vi "X_gConstraintsFun.vi"() -> (0 "constraints cluster":T1)   [LabVIEW 2019]
panel:
  in  "Ts":dbl=0.001
  in  "w0":dbl=1.0
  in  "weight":dbl[](array[numeric])=[1e-06, 1e-06, 1e-06, 1e-06, 1e-06, 1e-06, 1e-06, 1e-06, 1e-06, 1e-06, 1e-06, 1e-06, 1e-06, 1e-06, 1e-06, 1e-06, 1e-06, 1e-06]
  out "gamma":cdb
  out "beta":cdb[](array[numeric])
  in  "Ki":dbl[](array[numeric])=[1000.0, 100.0, 10.0, 1.4, 0.831, 0.35, 0.143, 0.139, 0.131, 0.113, 0.102, 0.092, 0.083, 0.0, 0.0, 0.0, 0.0, 0.0]
  out "OmegaC":dbl[](array[numeric])
  in  "freq(Hz)":dbl[](array[numeric])=[0.1, 1.0, 10.0, 100.0, 325.0, 500.0, 700.0, 1000.0, 1322.0, 1800.0, 2200.0, 2600.0, 3000.0, 0.0, 0.0, 0.0, 0.0, 0.0]
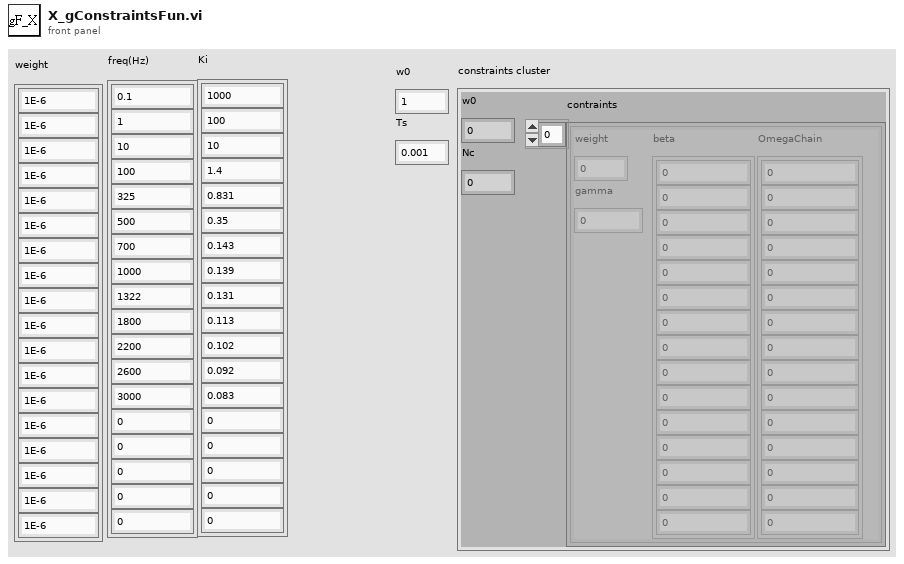
[diagram p1: front panel]
types:
  T1 = cluster{"w0":dbl, "contraints":cluster{"beta":dbl[], "gamma":dbl, "OmegaChain":dbl[], "weight":dbl}[], "Nc":i32}
  T2 = cluster{"v2p.num":dbl[], ".v2p.den":dbl[], "N.num":dbl[], "M.num":dbl[], "X.num":dbl[], "W.num":dbl[], "N.den":dbl[], "W.den":dbl[], "M.den":dbl[], "X.den":dbl[]}
  T3 = cluster{"beta":dbl[], "gamma":dbl, "OmegaChain":dbl[], "weight":dbl}
  T4 = cluster{"v2p":cdb, "N":cdb, "M":cdb, ".X":cdb, "W":cdb}
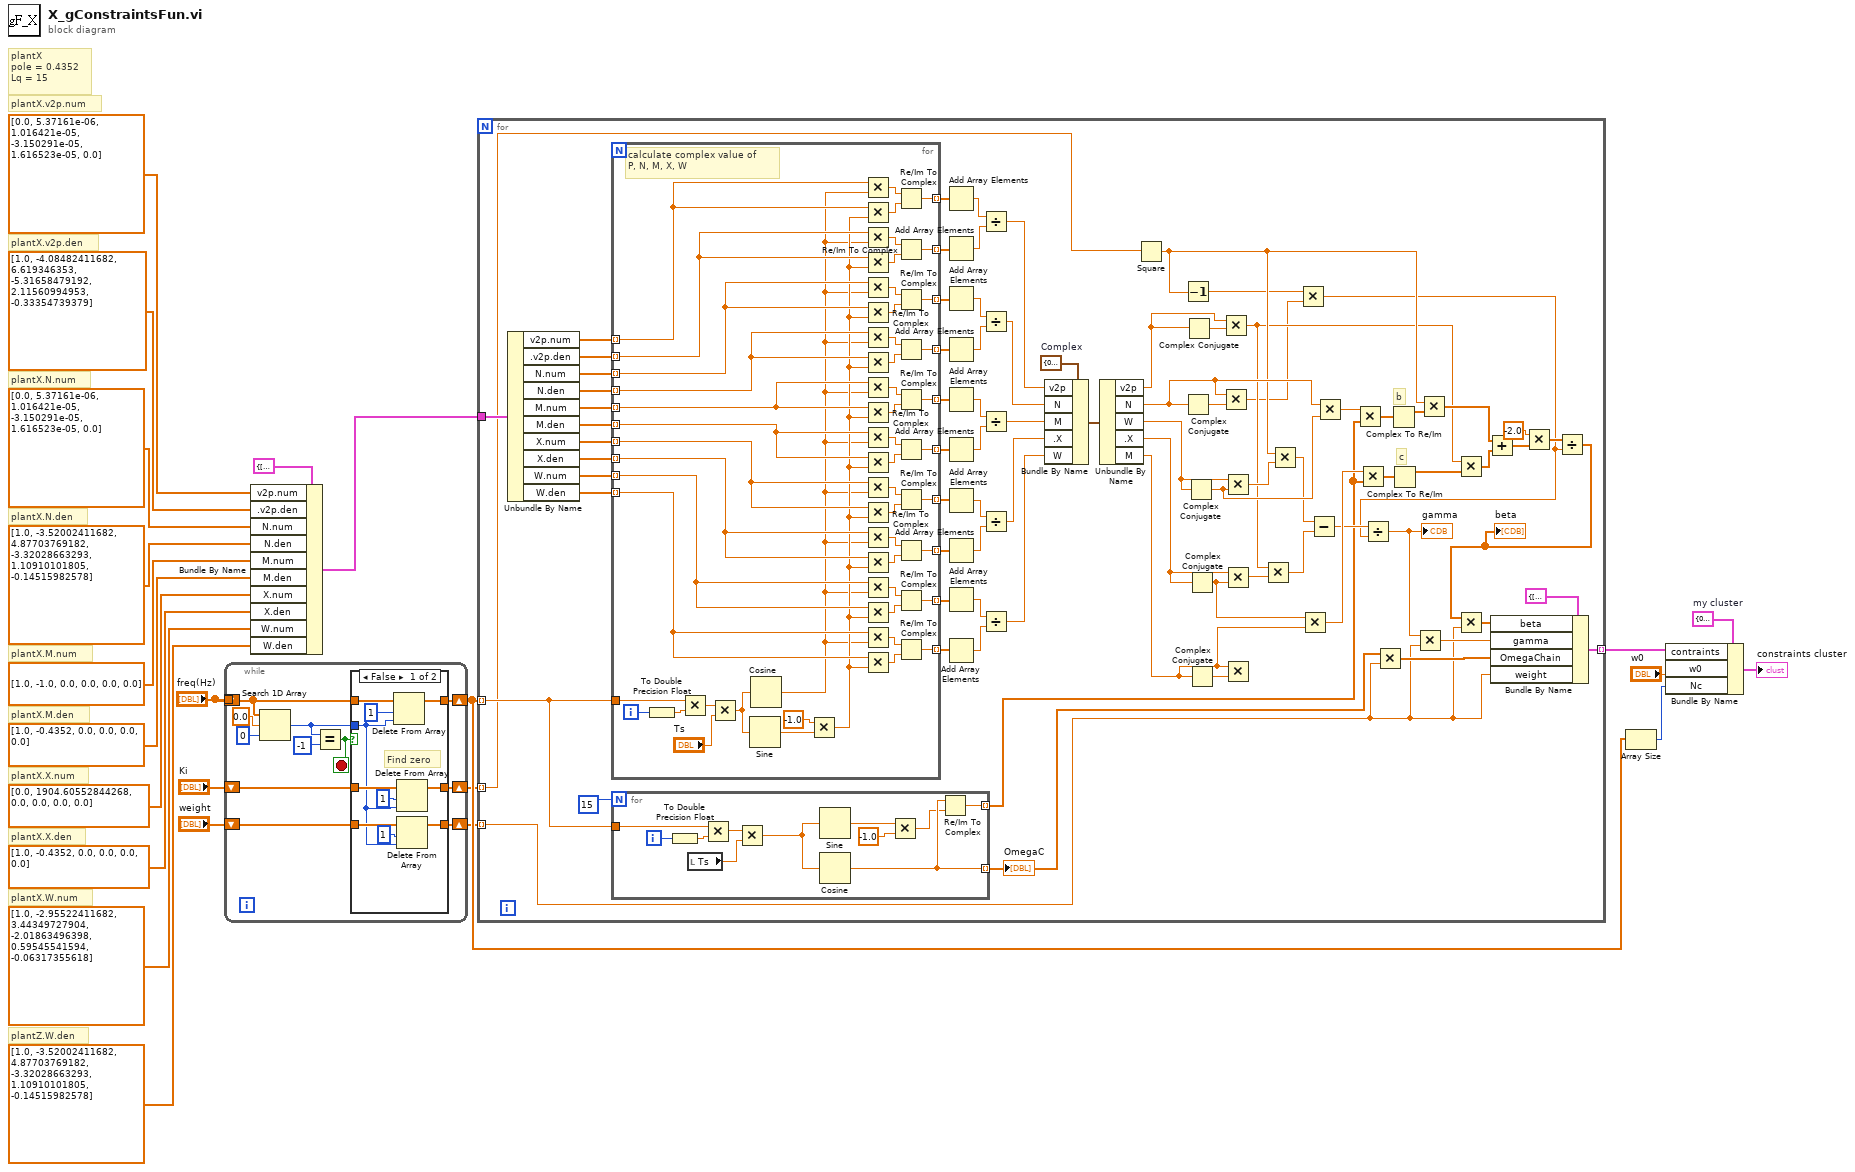
[diagram p0: block diagram]
diagram:
  w21 = T1 {"w0"=0.0, "contraints"=[], "Nc"=0}  # my cluster
  # "plantX.N.den"
  # "plantZ.W.den"
  # "plantX.M.den"
  # "plantX.X.den"
  # "plantX\npole = 0.4352\nLq = 15"
  # "plantX.W.num"
  # "plantX.X.num"
  # "plantX.M.num"
  # "plantX.N.num"
  # "plantX.v2p.den"
  # "plantX.v2p.num"
  n1 = while {
    shift-right: [w29] -> w5
    shift-left: "freq(Hz)" -> [w28]
    tunnel: "freq(Hz)" -> [_]
    shift-right: [w24] -> w2
    shift-left: "Ki" -> [w26]
    shift-right: [w25] -> w1
    shift-left: "weight" -> [w27]
    stop <- w30 stop-if-true
    n2 = Search 1D Array(1D array=w28, element=0.0, start index (0)=0) -> (index of element=w31:i32)
    n3 = Equal?(x=w31, y=-1) -> (x = y?=w30:bool)
    n4 = case shown="False" w30 {
      tunnel: w31 -> [w35 _]
      tunnel: w28 -> [w43 w47]
      tunnel: [w42 w47] -> w29
      tunnel: w26 -> [w39 w46]
      tunnel: w27 -> [w38 w45]
      tunnel: [w37 w45] -> w25
      tunnel: [w36 w46] -> w24
      frame False {
        # "Find zero"
        n5 = Delete From Array(array=w43, length=1, index=w35) -> (array with subset deleted=w42:dbl[])  [unwired: 1 out]
        n6 = Delete From Array(array=w39, length=1, index=w35) -> (array with subset deleted=w36:dbl[])  [unwired: 1 out]
        n7 = Delete From Array(array=w38, length=1, index=w35) -> (array with subset deleted=w37:dbl[])  [unwired: 1 out]
      }
      frame True {
        # "not find zero"
      }
    }
  }
  n8 = Bundle By Name(cluster=T2 {"v2p.num"=[0.0, 1.946435e-05, -4.19161e-05, 3.029095e-05, -7.40278e-06, 0.0], ".v2p.den"=[1.0, -4.44700230387, 7.99839085488, -7.28252340102, 3.36004265435, -0.62890780434], "N.num"=[0.0, 1.946435e-05, -4.19161e-05, 3.029095e-05, -7.40278e-06, 0.0], "M.num"=[1.0, -1.0], "X.num"=[0.0, 1260.742668649], "W.num"=[1.0, -3.43740230387, 4.74858083222, -3.28268820621, 1.12905179105, -0.15422268366], "N.den"=[0.0, 1.946435e-05, -4.19161e-05, 3.029095e-05, -7.40278e-06, 0.0], "W.den"=[1.0, -3.43740230387, 4.74858083222, -3.28268820621, 1.12905179105, -0.15422268366], "M.den"=[1.0, -1.0], "X.den"=[0.0, 1260.742668649]}, "v2p.num"=dbl[] [0.0, 5.37161e-06, 1.016421e-05, -3.150291e-05, 1.616523e-05, 0.0], ".v2p.den"=dbl[] [1.0, -4.08482411682, 6.619346353, -5.31658479192, 2.11560994953, -0.33354739379], "N.num"=dbl[] [0.0, 5.37161e-06, 1.016421e-05, -3.150291e-05, 1.616523e-05, 0.0], "N.den"=dbl[] [1.0, -3.52002411682, 4.87703769182, -3.32028663293, 1.10910101805, -0.14515982578], "M.num"=dbl[] [1.0, -1.0, 0.0, 0.0, 0.0, 0.0], "M.den"=dbl[] [1.0, -0.4352, 0.0, 0.0, 0.0, 0.0], "X.num"=dbl[] [0.0, 1904.60552844268, 0.0, 0.0, 0.0, 0.0], "X.den"=dbl[] [1.0, -0.4352, 0.0, 0.0, 0.0, 0.0], "W.num"=dbl[] [1.0, -2.95522411682, 3.44349727904, -2.01863496398, 0.59545541594, -0.06317355618], "W.den"=dbl[] [1.0, -3.52002411682, 4.87703769182, -3.32028663293, 1.10910101805, -0.14515982578]) -> (w22:T2)
  n9 = for {
    tunnel: w22 -> [w128]
    tunnel: [w86] -> w8 mode=indexing
    tunnel: w5 -> [w52] mode=indexing
    tunnel: w2 -> [w51] mode=indexing
    tunnel: w1 -> [w48] mode=indexing
    w121 = T4 {"v2p"=0.0+0.0i, "N"=0.0+0.0i, "M"=0.0+0.0i, ".X"=0.0+0.0i, "W"=0.0+0.0i}  # Complex
    # "c"
    # "b"
    n10 = Unbundle By Name(w128) -> ("v2p.num"=w122:dbl[], ".v2p.den"=w123:dbl[], "N.num"=w124:dbl[], "N.den"=w125:dbl[], "M.num"=w126:dbl[], "M.den"=w127:dbl[], "X.num"=w80:dbl[], "X.den"=w79:dbl[], "W.num"=w78:dbl[], "W.den"=w77:dbl[])
    n11 = for {
      tunnel: w127 -> [w169] mode=indexing
      tunnel: w126 -> [w170] mode=indexing
      tunnel: w125 -> [w171] mode=indexing
      tunnel: w124 -> [w172] mode=indexing
      tunnel: w123 -> [w173] mode=indexing
      tunnel: w122 -> [w174] mode=indexing
      tunnel: w52 -> [w177]
      tunnel: w80 -> [w147] mode=indexing
      tunnel: w79 -> [w146] mode=indexing
      tunnel: w78 -> [w143] mode=indexing
      tunnel: w77 -> [w142] mode=indexing
      tunnel: [w139] -> w76 mode=indexing
      tunnel: [w138] -> w75 mode=indexing
      tunnel: [w137] -> w74 mode=indexing
      tunnel: [w136] -> w73 mode=indexing
      tunnel: [w135] -> w72 mode=indexing
      tunnel: [w134] -> w71 mode=indexing
      tunnel: [w133] -> w70 mode=indexing
      tunnel: [w132] -> w69 mode=indexing
      tunnel: [w131] -> w68 mode=indexing
      tunnel: [w130] -> w67 mode=indexing
      i -> [w179]
      # "calculate complex value of\nP, N, M, X, W"
      n12 = To Double Precision Float(number=w179) -> (double precision float=w178:dbl)
      n13 = Multiply(x=w177, y=w178) -> (x*y=w168:dbl)
      n14 = Multiply(x=w168, y="Ts") -> (x*y=w167:dbl)
      n15 = Sine(x=w167) -> (sin(x)=w176:dbl)
      n16 = Cosine(x=w167) -> (cos(x)=w140:dbl)
      n17 = Multiply(x=-1.0, y=w176) -> (x*y=w141:dbl)
      n18 = Multiply(x=w174, y=w140) -> (x*y=w165:dbl)
      n19 = Multiply(x=w174, y=w141) -> (x*y=w164:dbl)
      n20 = Multiply(x=w173, y=w140) -> (x*y=w163:dbl)
      n21 = Multiply(x=w173, y=w141) -> (x*y=w162:dbl)
      n22 = Multiply(x=w172, y=w140) -> (x*y=w161:dbl)
      n23 = Multiply(x=w172, y=w141) -> (x*y=w160:dbl)
      n24 = Multiply(x=w171, y=w140) -> (x*y=w159:dbl)
      n25 = Multiply(x=w171, y=w141) -> (x*y=w158:dbl)
      n26 = Multiply(x=w170, y=w140) -> (x*y=w157:dbl)
      n27 = Multiply(x=w170, y=w141) -> (x*y=w156:dbl)
      n28 = Multiply(x=w169, y=w140) -> (x*y=w155:dbl)
      n29 = Multiply(x=w169, y=w141) -> (x*y=w154:dbl)
      n30 = Multiply(x=w147, y=w140) -> (x*y=w153:dbl)
      n31 = Multiply(x=w147, y=w141) -> (x*y=w152:dbl)
      n32 = Multiply(x=w146, y=w140) -> (x*y=w151:dbl)
      n33 = Multiply(x=w146, y=w141) -> (x*y=w150:dbl)
      n34 = Multiply(x=w143, y=w140) -> (x*y=w149:dbl)
      n35 = Multiply(x=w143, y=w141) -> (x*y=w148:dbl)
      n36 = Multiply(x=w142, y=w140) -> (x*y=w145:dbl)
      n37 = Multiply(x=w142, y=w141) -> (x*y=w144:dbl)
      n38 = Re/Im To Complex(1:w164, 2:w165) -> (0:w139:cdb)
      n39 = Re/Im To Complex(1:w162, 2:w163) -> (0:w138:cdb)
      n40 = Re/Im To Complex(1:w160, 2:w161) -> (0:w137:cdb)
      n41 = Re/Im To Complex(1:w158, 2:w159) -> (0:w136:cdb)
      n42 = Re/Im To Complex(1:w156, 2:w157) -> (0:w135:cdb)
      n43 = Re/Im To Complex(1:w154, 2:w155) -> (0:w134:cdb)
      n44 = Re/Im To Complex(1:w152, 2:w153) -> (0:w133:cdb)
      n45 = Re/Im To Complex(1:w150, 2:w151) -> (0:w132:cdb)
      n46 = Re/Im To Complex(1:w148, 2:w149) -> (0:w131:cdb)
      n47 = Re/Im To Complex(1:w144, 2:w145) -> (0:w130:cdb)
    }
    n48 = for {
      N: 15 -> [_]
      tunnel: w52 -> [w189]
      tunnel: [w185] -> w49 mode=indexing
      tunnel: [w183] -> w50 mode=indexing
      i -> [w190]
      n49 = To Double Precision Float(number=w190) -> (double precision float=w188:dbl)
      n50 = local read "Ts"() -> (w180:dbl)
      n51 = Multiply(x=w189, y=w188) -> (x*y=w181:dbl)
      n52 = Multiply(x=w181, y=w180) -> (x*y=w182:dbl)
      n53 = Sine(x=w182) -> (sin(x)=w187:dbl)
      n54 = Cosine(x=w182) -> (cos(x)=w185:dbl)
      n55 = Multiply(x=w187, y=-1.0) -> (x*y=w184:dbl)
      n56 = Re/Im To Complex(1:w184, 2:w185) -> (0:w183:cdb)
    }
    "OmegaC" <- w49
    n57 = Add Array Elements(numeric array=w76) -> (sum=w66:cdb)
    n58 = Add Array Elements(numeric array=w75) -> (sum=w65:cdb)
    n59 = Add Array Elements(numeric array=w74) -> (sum=w64:cdb)
    n60 = Add Array Elements(numeric array=w73) -> (sum=w63:cdb)
    n61 = Add Array Elements(numeric array=w72) -> (sum=w62:cdb)
    n62 = Add Array Elements(numeric array=w71) -> (sum=w61:cdb)
    n63 = Add Array Elements(numeric array=w70) -> (sum=w60:cdb)
    n64 = Add Array Elements(numeric array=w69) -> (sum=w59:cdb)
    n65 = Add Array Elements(numeric array=w68) -> (sum=w58:cdb)
    n66 = Add Array Elements(numeric array=w67) -> (sum=w57:cdb)
    n67 = Divide(x=w66, y=w65) -> (x/y=w120:cdb)
    n68 = Divide(x=w64, y=w63) -> (x/y=w56:cdb)
    n69 = Divide(x=w62, y=w61) -> (x/y=w55:cdb)
    n70 = Divide(x=w60, y=w59) -> (x/y=w54:cdb)
    n71 = Divide(x=w58, y=w57) -> (x/y=w53:cdb)
    n72 = Bundle By Name(cluster=w121, "v2p"=w120, "N"=w56, "M"=w55, ".X"=w54, "W"=w53) -> (w89:T4)
    n73 = Unbundle By Name(w89) -> ("v2p"=w114:cdb, "N"=w106:cdb, "W"=w111:cdb, ".X"=w110:cdb, "M"=w109:cdb)
    n74 = Square(x=w51) -> (x^2=w99:dbl)
    n75 = Decrement(x=w99) -> (x-1=w93:dbl)
    n76 = Complex Conjugate(1:w106) -> (0:w113:cdb)
    n77 = Complex Conjugate(1:w114) -> (0:w115:cdb)
    n78 = Complex Conjugate(1:w111) -> (0:w107:cdb)
    n79 = Complex Conjugate(1:w110) -> (0:w108:cdb)
    n80 = Complex Conjugate(1:w109) -> (0:w112:cdb)
    n81 = Multiply(x=w114, y=w115) -> (x*y=w96:cdb)
    n82 = Multiply(x=w106, y=w113) -> (x*y=w92:cdb)
    n83 = Multiply(x=w111, y=w107) -> (x*y=w98:cdb)
    n84 = Multiply(x=w110, y=w108) -> (x*y=w97:cdb)
    n85 = Multiply(x=w109, y=w112) -> ()  [unwired: 1 out]
    n86 = Multiply(x=w96, y=w97) -> (x*y=w94:cdb)
    n87 = Multiply(x=w99, y=w98) -> (x*y=w95:cdb)
    n88 = Multiply(x=w93, y=w92) -> (x*y=w88:cdb)
    n89 = Multiply(x=w108, y=w109) -> (x*y=w119:cdb)
    n90 = Subtract(x=w95, y=w94) -> (x-y=w90:cdb)
    n91 = Multiply(x=w106, y=w107) -> (x*y=w117:cdb)
    n92 = Multiply(x=w117, y=w50) -> (x*y=w116:cdb[])
    n93 = Multiply(x=w119, y=w50) -> (x*y=w118:cdb[])
    n94 = Divide(x=w90, y=w88) -> (x/y=w83:cdb)
    "gamma" <- w83
    n95 = Multiply(x=w49, y=w48) -> (x*y=w85:dbl[])
    n96 = Complex To Re/Im(x + iy=w116) -> (x=w105:dbl[])  [unwired: 1 out]
    n97 = Complex To Re/Im(x + iy=w118) -> (x=w104:dbl[])  [unwired: 1 out]
    n98 = Multiply(x=w83, y=w48) -> (x*y=w84:cdb)
    n99 = Multiply(x=w99, y=w105) -> (x*y=w103:dbl[])
    n100 = Multiply(x=w96, y=w104) -> (x*y=w102:cdb[])
    n101 = Add(x=w103, y=w102) -> (x+y=w101:cdb[])
    n102 = Multiply(x=-2.0, y=w101) -> (x*y=w91:cdb[])
    n103 = Divide(x=w91, y=w88) -> (x/y=w81:cdb[])
    "beta" <- w81
    n104 = Multiply(x=w81, y=w48) -> (x*y=w82:cdb[])
    n105 = Bundle By Name(cluster=T3 {"beta"=[], "gamma"=0.0, "OmegaChain"=[], "weight"=0.0}, "beta"=w82, "gamma"=w84, "OmegaChain"=w85, "weight"=w48) -> (w86:T3)
  }
  n106 = Array Size(array=w5) -> (size(s)=w9:i32)
  n107 = Bundle By Name(cluster=w21, "contraints"=w8, "w0"="w0", "Nc"=w9) -> (→"constraints cluster":T1)
